vi "Boiler Controller.vi"(8 "error in (no error)":errorcluster, 9 "Controller Configuration Data":T1, 10 "Notifiers":T2, 11 "All Message Queues":T3) -> (0 "error out":errorcluster)   [LabVIEW 2017, in "Controller.lvlib"]
uses:
  Controller.lvlib
  support/Message Queue/All Message Queues.ctl
  support/Message Queue/Message Cluster.ctl
  support/Notifieres/Notifiers.ctl
  Controller Configuration.ctl
  controls/MHL UI Data.ctl
  controls/MHL Status.ctl
  support/Boiler System Globals.vi
  <vilib>/Utility/error.llb/Error Cluster From Error Code.vi
  <vilib>/ErrorRing/Error Ring.xnode
  support/Message Queue/Message Queue.lvlib
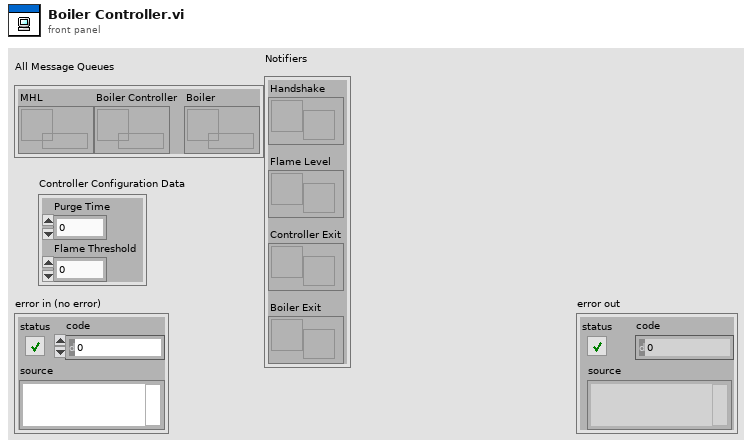
[diagram p1: front panel]
types:
  T1 = typedef "Controller.lvlib/Controller Configuration.ctl" = cluster{"Purge Time":u32, "Flame Threshold":u32}
  T2 = typedef "Notifiers.ctl" = cluster{"Handshake":refnum<notifier>, "Flame Level":refnum<notifier>, "Controller Exit":refnum<notifier>, "Boiler Exit":refnum<notifier>}
  T3 = typedef "Message Queue.lvlib/All Message Queues.ctl" = cluster{"MHL":refnum<queue>, "Boiler Controller":refnum<queue>, "Boiler":refnum<queue>}
  T4 = enum16{"open", "replace", "create", "open or create", "replace or create", "replace or create with confirmation"}
  T5 = typedef "MHL Status.ctl" = enum16{"Lockout", "Ready", "Pre-Purge", "Pre-Purge Complete", "Pilot On", "Boiler Running", "Shutdown", "Purge"}
  T6 = typedef "MHL UI Data.ctl" = cluster{"Status":string, "Fuel Control Valve":u32, "Primary Fan":bool, "Pilot Gas Valve":bool, "Pilot":bool, "Forced Draft Fan":bool, "MHL Status":T5}
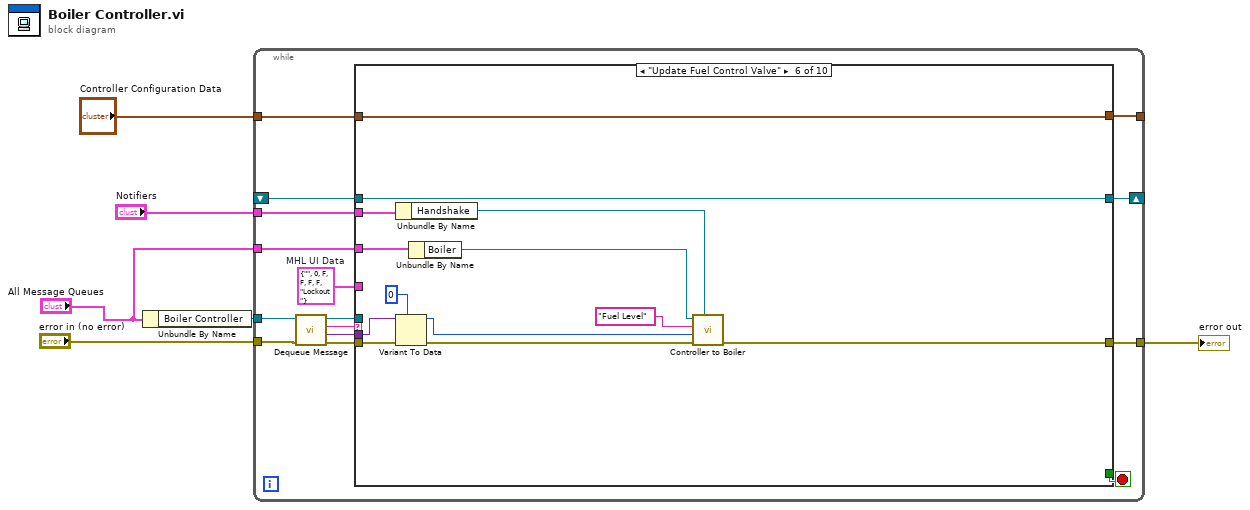
[diagram p0: block diagram]
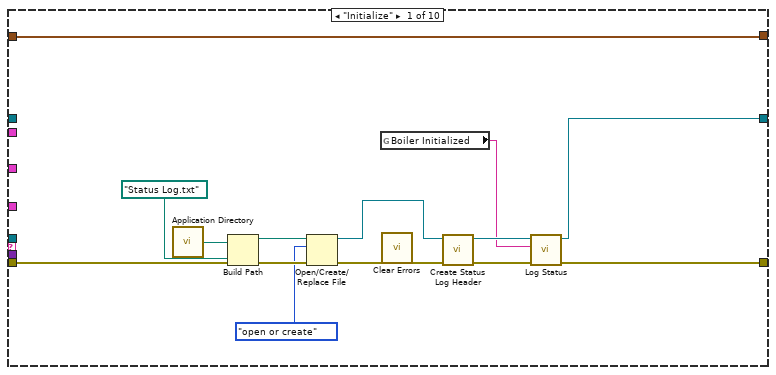
[diagram p2: hidden frame]
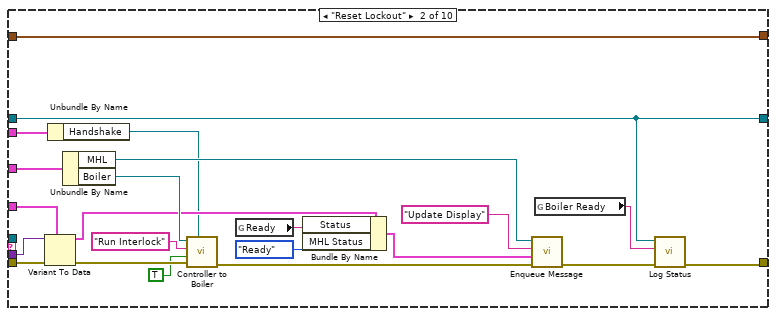
[diagram p3: hidden frame]
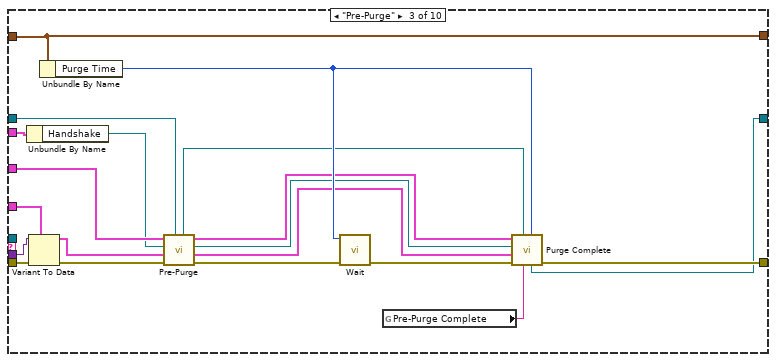
[diagram p4: hidden frame]
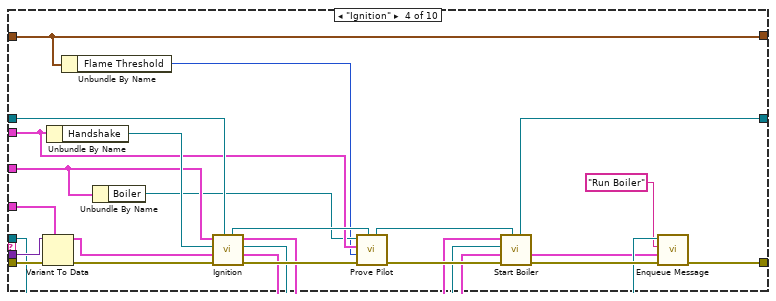
[diagram p5: hidden frame]
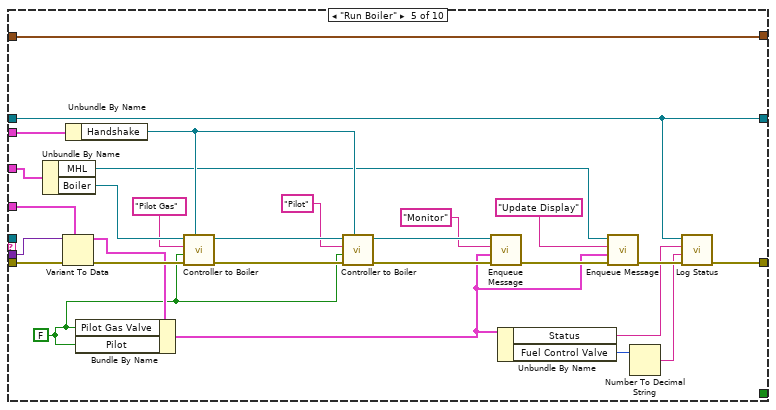
[diagram p6: hidden frame]
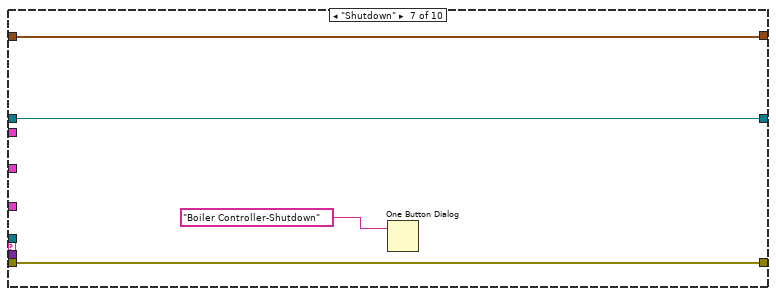
[diagram p7: hidden frame]
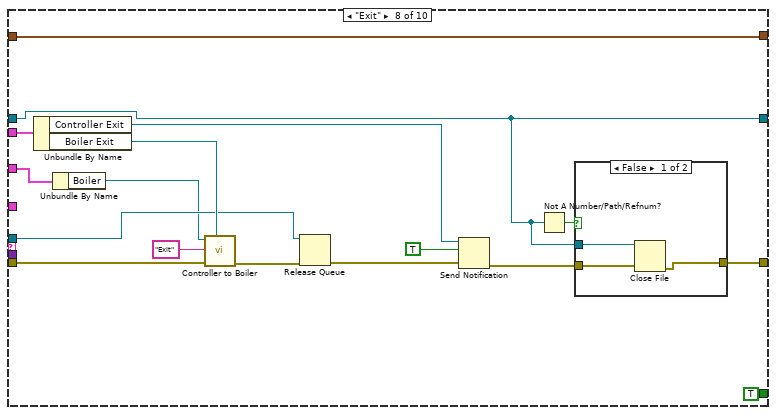
[diagram p8: hidden frame]
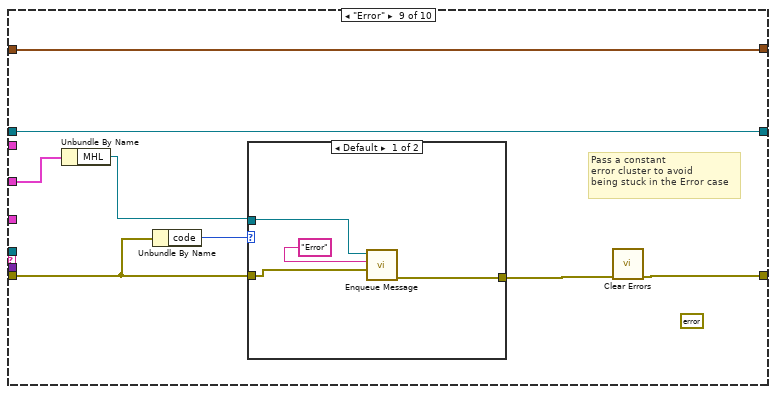
[diagram p10: hidden frame]
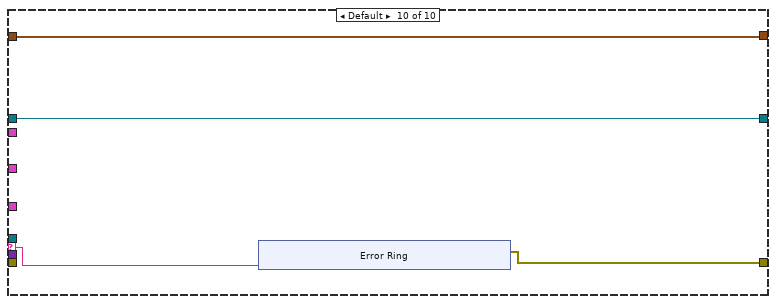
[diagram p12: hidden frame]
diagram:
  n1 = Unbundle By Name("All Message Queues") -> ("Boiler Controller"=w6:refnum<queue>)
  n2 = while {
    tunnel: w6 -> [w21]
    tunnel: "error in (no error)" -> [w20]
    tunnel: [w18] -> w4
    tunnel: "Notifiers" -> [w14]
    shift-right: [w13] -> _
    shift-left: _ -> [w12]
    tunnel: "All Message Queues" -> [w9]
    tunnel: "Controller Configuration Data" -> [w8]
    tunnel: [w7] -> _
    stop <- w15 stop-if-true
    w10 = T6 {"Status"="", "Fuel Control Valve"=0, "Primary Fan"=FALSE, "Pilot Gas Valve"=FALSE, "Pilot"=FALSE, "Forced Draft Fan"=FALSE, "MHL Status"=enum."Lockout"}  # MHL UI Data
    n3 = call "Dequeue Message.vi"("error in (no error)"=w20, "Message Queue"=w21) -> ("error out"=w19:errorcluster, "Message Data"=w11:variant, "Message"=w17:string, "dup Message Queue"=w16:refnum<queue>)  [unwired: 6 in]
    n4 = case shown="\"Update Fuel Control Valve\"" w17 {
      selector: w17 -> [_ _ _ _ _ _ _ _ _ w185]
      tunnel: w19 -> [w28 w57 w77 w96 w129 w140 w147 w162 w176 _]
      tunnel: [w27 w40 w65 w81 w110 w141 w147 w153 w173 w184] -> w18
      tunnel: w16 -> [_ _ _ w80 _ _ _ w155 _ _]
      tunnel: [_ _ _ _ _ _ _ TRUE _ _] -> w15
      tunnel: w14 -> [_ w43 w73 w87 w123 w133 _ w163 _ _]
      tunnel: [w31 w39 w58 w99 w103 w143 w145 w151 w172 w183] -> w13
      tunnel: w12 -> [_ w39 w71 w100 w103 w143 w145 w151 w172 w183]
      tunnel: w11 -> [_ w56 w70 w93 w112 w138 _ _ _ _]
      tunnel: w10 -> [_ w55 w75 w94 w113 _ _ _ _ _]
      tunnel: w9 -> [_ w54 w74 w86 w124 w134 _ w150 w171 _]
      tunnel: w8 -> [w22 w36 w67 w84 w130 w142 w144 w148 w169 w182]
      tunnel: [w22 w36 w67 w84 w130 w142 w144 w148 w169 w182] -> w7
      frame "Initialize" {
        n5 = call <vilib>:"Application Directory.vi"() -> ("Application Directory"=w30:path)
        n6 = Build Path(base path=w30, name or relative path=path "Status Log.txt") -> (appended path=w35:path)
        n7 = Open/Create/Replace File(file path (use dialog)=w35, error in=w28, operation (0:open)=T4."open or create") -> (refnum out=w34:refnum<file>, error out=w26:errorcluster)  [unwired: 3 in, 1 out]
        n8 = global read "Boiler System Globals.vi" "Boiler Initialized"() -> (w24:string)
        n9 = call <vilib>:"Clear Errors.vi"("error in (no error)"=w26) -> ("error out"=w25:errorcluster)  [unwired: 5 in, 1 out]
        n10 = call "Create Status Log Header.vi"("error in"=w25, "Log File Refnum in"=w34) -> ("error out"=w32:errorcluster, "Log File Refnum out"=w33:refnum<file>)  [unwired: 8 in]
        n11 = call "Log Status.vi"("error in"=w32, "Event String"=w24, "Log File Refnum In"=w33) -> ("error out"=w27:errorcluster, "Log File Refnum Out"=w31:refnum<file>)  [unwired: 7 in]
      }
      frame "Reset Lockout" {
        n12 = Variant To Data(error in=w57, type=w55, Variant=w56) -> (data=w50:T6, error out=w47:errorcluster)
        n13 = Unbundle By Name(w43) -> ("Handshake"=w42:refnum<notifier>)
        n14 = Unbundle By Name(w54) -> ("MHL"=w52:refnum<queue>, "Boiler"=w53:refnum<queue>)
        n15 = call "Controller to Boiler.vi"("Notifier"=w42, "error in"=w47, "Message Data"=TRUE, "Message"="Run Interlock", "Boiler Queue in"=w53) -> ("error out"=w46:errorcluster)  [unwired: 4 in, 2 out]
        n16 = global read "Boiler System Globals.vi" "Ready"() -> (w49:string)
        n17 = Bundle By Name(cluster=w50, "Status"=w49, "MHL Status"=MHL_Status."Ready") -> (w48:T6)
        n18 = call "Enqueue Message.vi"("error in (no error)"=w46, "Message Data"=w48, "Message"="Update Display", "Message Queue"=w52) -> ("error out"=w41:errorcluster)  [unwired: 6 in, 1 out]
        n19 = global read "Boiler System Globals.vi" "Boiler Ready"() -> (w38:string)
        n20 = call "Log Status.vi"("error in"=w41, "Event String"=w38, "Log File Refnum In"=w39) -> ("error out"=w40:errorcluster)  [unwired: 7 in, 1 out]
      }
      frame "Pre-Purge" {
        n21 = Unbundle By Name(w73) -> ("Handshake"=w72:refnum<notifier>)
        n22 = Variant To Data(error in=w77, type=w75, Variant=w70) -> (data=w69:T6, error out=w76:errorcluster)
        n23 = Unbundle By Name(w67) -> ("Purge Time"=w64:u32)
        n24 = call "Pre-Purge.vi"("Log File Refnum in"=w71, "error in"=w76, "UI Data in"=w69, "Handshake Notifier in"=w72, "Message Queues in"=w74) -> ("error out"=w68:errorcluster, "UI Data out"=w61:T6, "Handshake Notifier out"=w62:refnum<notifier>, "Message Queues out"=w63:T3, "Log File Refnum out"=w59:refnum<file>)  [unwired: 2 in]
        n25 = call "Wait.vi"("error in"=w68, "Purge Time (s)"=w64) -> ("error out"=w66:errorcluster)  [unwired: 9 in]
        n26 = global read "Boiler System Globals.vi" "Pre-Purge Complete"() -> (w60:string)
        n27 = call "Purge Complete.vi"("Purge Time"=w64, "Status"=w60, "Log File Refnum in"=w59, "error in"=w66, "UI Data in"=w61, "Handshake Notifier in"=w62, "Message Queues in"=w63) -> ("error out"=w65:errorcluster, "Log File Refnum out"=w58:refnum<file>)  [unwired: 3 out]
      }
      frame "Ignition" {
        n28 = Variant To Data(error in=w96, type=w94, Variant=w93) -> (data=w90:T6, error out=w95:errorcluster)
        n29 = Unbundle By Name(w87) -> ("Handshake"=w91:refnum<notifier>)
        n30 = Unbundle By Name(w84) -> ("Flame Threshold"=w83:u32)
        n31 = Unbundle By Name(w86) -> ("Boiler"=w85:refnum<queue>)
        n32 = call "Ignition.vi"("Log File Refnum in"=w100, "error in"=w95, "UI Data in"=w90, "Handshake Notifier in"=w91, "Message Queues in"=w86) -> ("error out"=w102:errorcluster, "UI Data out"=w88:T6, "Handshake Notifier out"=w89:refnum<notifier>, "Message Queues out"=w92:T3, "Log File Refnum out"=w97:refnum<file>)  [unwired: 2 in]
        n33 = call "Prove Pilot.vi"("Log File Refnum in"=w97, "error in"=w102, "Flame Threshold"=w83, "Notifiers in"=w87, "Boiler Queue in"=w85) -> ("error out"=w101:errorcluster, "Log File Refnum out"=w98:refnum<file>)  [unwired: 3 in, 2 out]
        n34 = call "Start Boiler.vi"("Log File Refnum in"=w98, "error in"=w101, "UI Data in"=w88, "Handshake Notifier in"=w89, "Message Queues in"=w92) -> ("error out"=w82:errorcluster, "UI Data out"=w79:T6, "Log File Refnum out"=w99:refnum<file>)  [unwired: 2 in, 2 out]
        n35 = call "Enqueue Message.vi"("error in (no error)"=w82, "Message Data"=w79, "Message"="Run Boiler", "Message Queue"=w80) -> ("error out"=w81:errorcluster)  [unwired: 6 in, 1 out]
      }
      frame "Run Boiler" {
        w108 = FALSE
        n36 = Unbundle By Name(w124) -> ("MHL"=w119:refnum<queue>, "Boiler"=w121:refnum<queue>)
        n37 = Variant To Data(error in=w129, type=w113, Variant=w112) -> (data=w109:T6, error out=w128:errorcluster)
        n38 = Unbundle By Name(w123) -> ("Handshake"=w122:refnum<notifier>)
        n39 = Bundle By Name(cluster=w109, "Pilot Gas Valve"=w108, "Pilot"=w108) -> (w107:T6)
        n40 = call "Controller to Boiler.vi"("Notifier"=w122, "error in"=w128, "Message Data"=w108, "Message"="Pilot Gas", "Boiler Queue in"=w121) -> ("error out"=w127:errorcluster, "Queue out"=w120:refnum<queue>)  [unwired: 4 in, 1 out]
        n41 = call "Controller to Boiler.vi"("Notifier"=w122, "error in"=w127, "Message Data"=w108, "Message"="Pilot", "Boiler Queue in"=w120) -> ("error out"=w126:errorcluster, "Queue out"=w118:refnum<queue>)  [unwired: 4 in, 1 out]
        n42 = call "Enqueue Message.vi"("error in (no error)"=w126, "Message Data"=w107, "Message"="Monitor", "Message Queue"=w118) -> ("error out"=w125:errorcluster)  [unwired: 6 in, 1 out]
        n43 = Unbundle By Name(w107) -> ("Status"=w105:string, "Fuel Control Valve"=w106:u32)
        n44 = call "Enqueue Message.vi"("error in (no error)"=w125, "Message Data"=w107, "Message"="Update Display", "Message Queue"=w119) -> ("error out"=w111:errorcluster)  [unwired: 6 in, 1 out]
        n45 = Number To Decimal String(number=w106) -> (decimal integer string=w104:string)  [unwired: 1 in]
        n46 = call "Log Status.vi"("error in"=w111, "Event Data String (-)"=w104, "Event String"=w105, "Log File Refnum In"=w103) -> ("error out"=w110:errorcluster)  [unwired: 6 in, 1 out]
      }
      frame "Update Fuel Control Valve" {
        n47 = Unbundle By Name(w133) -> ("Handshake"=w131:refnum<notifier>)
        n48 = Variant To Data(error in=w140, type=0, Variant=w138) -> (data=w136:i32, error out=w139:errorcluster)
        n49 = Unbundle By Name(w134) -> ("Boiler"=w132:refnum<queue>)
        n50 = call "Controller to Boiler.vi"("Notifier"=w131, "error in"=w139, "Message Data"=w136, "Message"="Fuel Level", "Boiler Queue in"=w132) -> ("error out"=w141:errorcluster)  [unwired: 4 in, 2 out]
      }
      frame "Shutdown" {
        n51 = One Button Dialog(message="Boiler Controller-Shutdown") -> ()  [unwired: 1 in, 1 out]
      }
      frame "Exit" {
        n52 = Unbundle By Name(w163) -> ("Controller Exit"=w157:refnum<notifier>, "Boiler Exit"=w160:refnum<notifier>)
        n53 = Unbundle By Name(w150) -> ("Boiler"=w149:refnum<queue>)
        n54 = call "Controller to Boiler.vi"("Notifier"=w160, "error in"=w162, "Message"="Exit", "Boiler Queue in"=w149) -> ("error out"=w161:errorcluster)  [unwired: 5 in, 2 out]
        n55 = Release Queue(queue=w155, error in (no error)=w161) -> (error out=w158:errorcluster)  [unwired: 1 in, 2 out]
        n56 = Send Notification(notification=TRUE, notifier=w157, error in (no error)=w158) -> (error out=w154:errorcluster)  [unwired: 1 out]
        n57 = Not A Number/Path/Refnum?(number/path/refnum=w151) -> (NaN/Path/Refnum?=w152:bool)
        n58 = case shown="False" w152 {
          tunnel: w154 -> [w167 w168]
          tunnel: [w166 w168] -> w153
          tunnel: w151 -> [w165 _]
          frame False {
            n59 = Close File(refnum=w165, error in=w167) -> (error out=w166:errorcluster)  [unwired: 1 out]
          }
          frame True {
          }
        }
      }
      frame "Error" {
        (unwired) errorcluster {"status"=FALSE, "code"=0, "source"=""} ("error constant")
        # "Pass a constant\nerror cluster to avoid\nbeing stuck in the Error case"
        n60 = Unbundle By Name(w171) -> ("MHL"=w170:refnum<queue>)
        n61 = Unbundle By Name(w176) -> ("code"=w175:i32)
        n62 = case shown="Default" w175 {
          tunnel: w170 -> [w180 _]
          tunnel: w176 -> [w178 w181]
          tunnel: [w177 w181] -> w174
          frame Default {
            n63 = call "Enqueue Message.vi"("Message Data"=w178, "Message"="Error", "Message Queue"=w180) -> ("error out"=w177:errorcluster)  [unwired: 7 in, 1 out]
          }
          frame 5000..5002 {
          }
        }
        n64 = call <vilib>:"Clear Errors.vi"("error in (no error)"=w174) -> ("error out"=w173:errorcluster)  [unwired: 5 in, 1 out]
      }
      frame Default {
        n65 = xnode "Error Ring"("parameter 0"=w185) -> ("error out"=w184:errorcluster)
      }
    }
  }
  "error out" <- w4
